vi "FiberWLCFruptCalc.vi"(9 "params in (all)":dbl[](array[numeric])=[0.0, 0.0, 6000.0, 50.0, 900.0, 197.0, 1.7, 0.3, 105.0, 80.0, 17.0, 5.0], 10 "tracename":string="E:\\users\\noort\\data\\270404\\_001.log") -> (1 "Channel data":dbl[][](array[numeric]), 2 "Channels":string[](array[string]), 3 "Lwrap (bp)":i16[](graph))   [LabVIEW 2018]
uses:
  <vilib>/Analysis/NI_AALBase.lvlib
panel:
  in  "Force treshold (pN)":dbl=5.0
  out "Lwrap (bp) 2":i32[](graph)
  out "F(z) Graph":cluster{"Data":dbl[], "Data":dbl[]}[](graph)
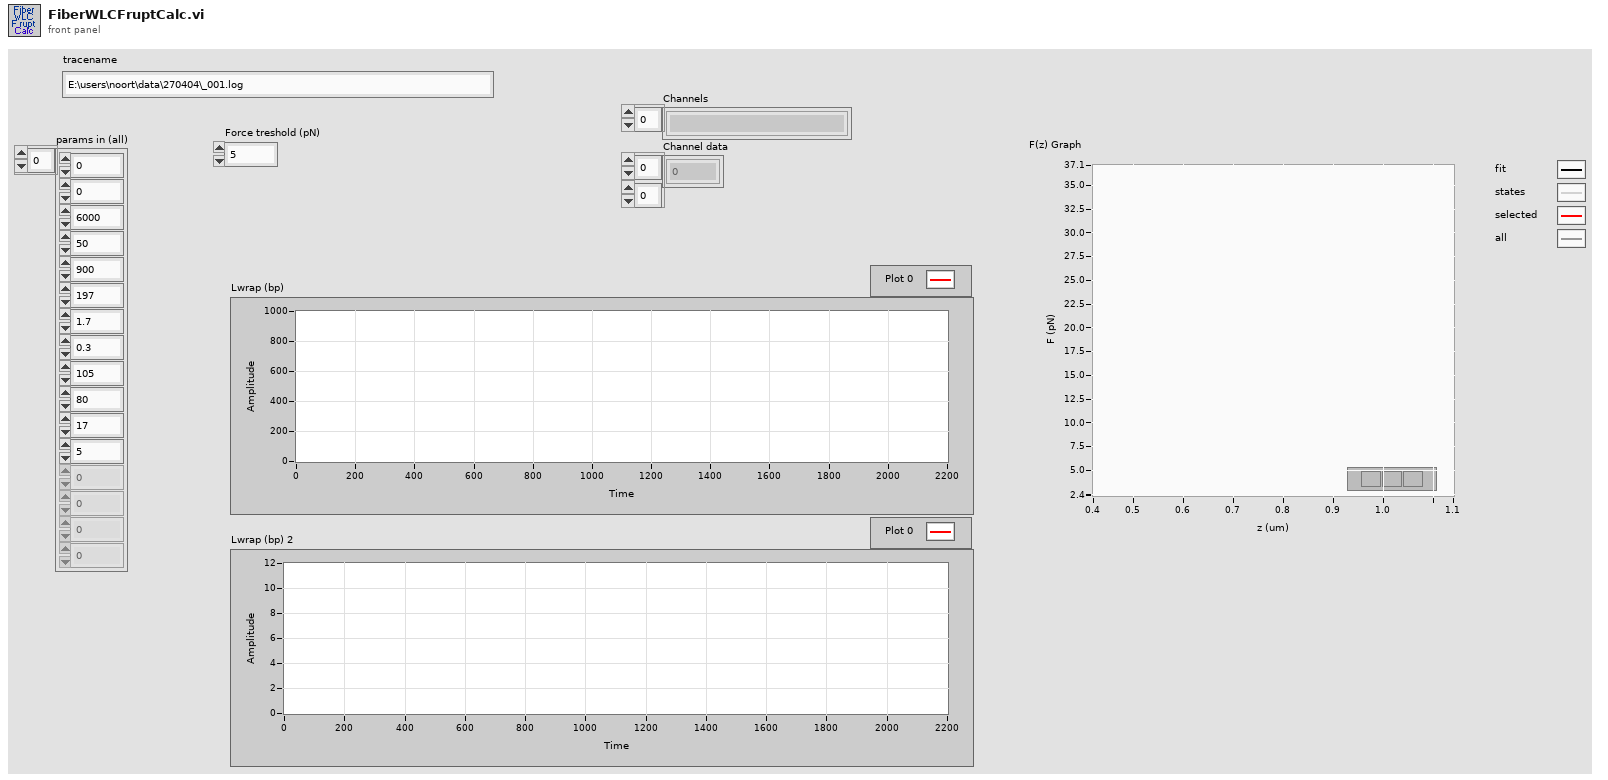
[diagram p1: front panel]
types:
  T1 = enum16{"Read", "Write", "Get channels", "Delete channels"}
  T2 = enum16{"Z0 (nm)", "dZ/dt (nm/s)", "L (bp)", "P (nm)", "S (pN)", "NRL (bp)", "NLD (nm)", "k (pN/nm)", "Lwrap1 (bp)", "Lwrap2 (bp)", "N4+N8", "N4"}
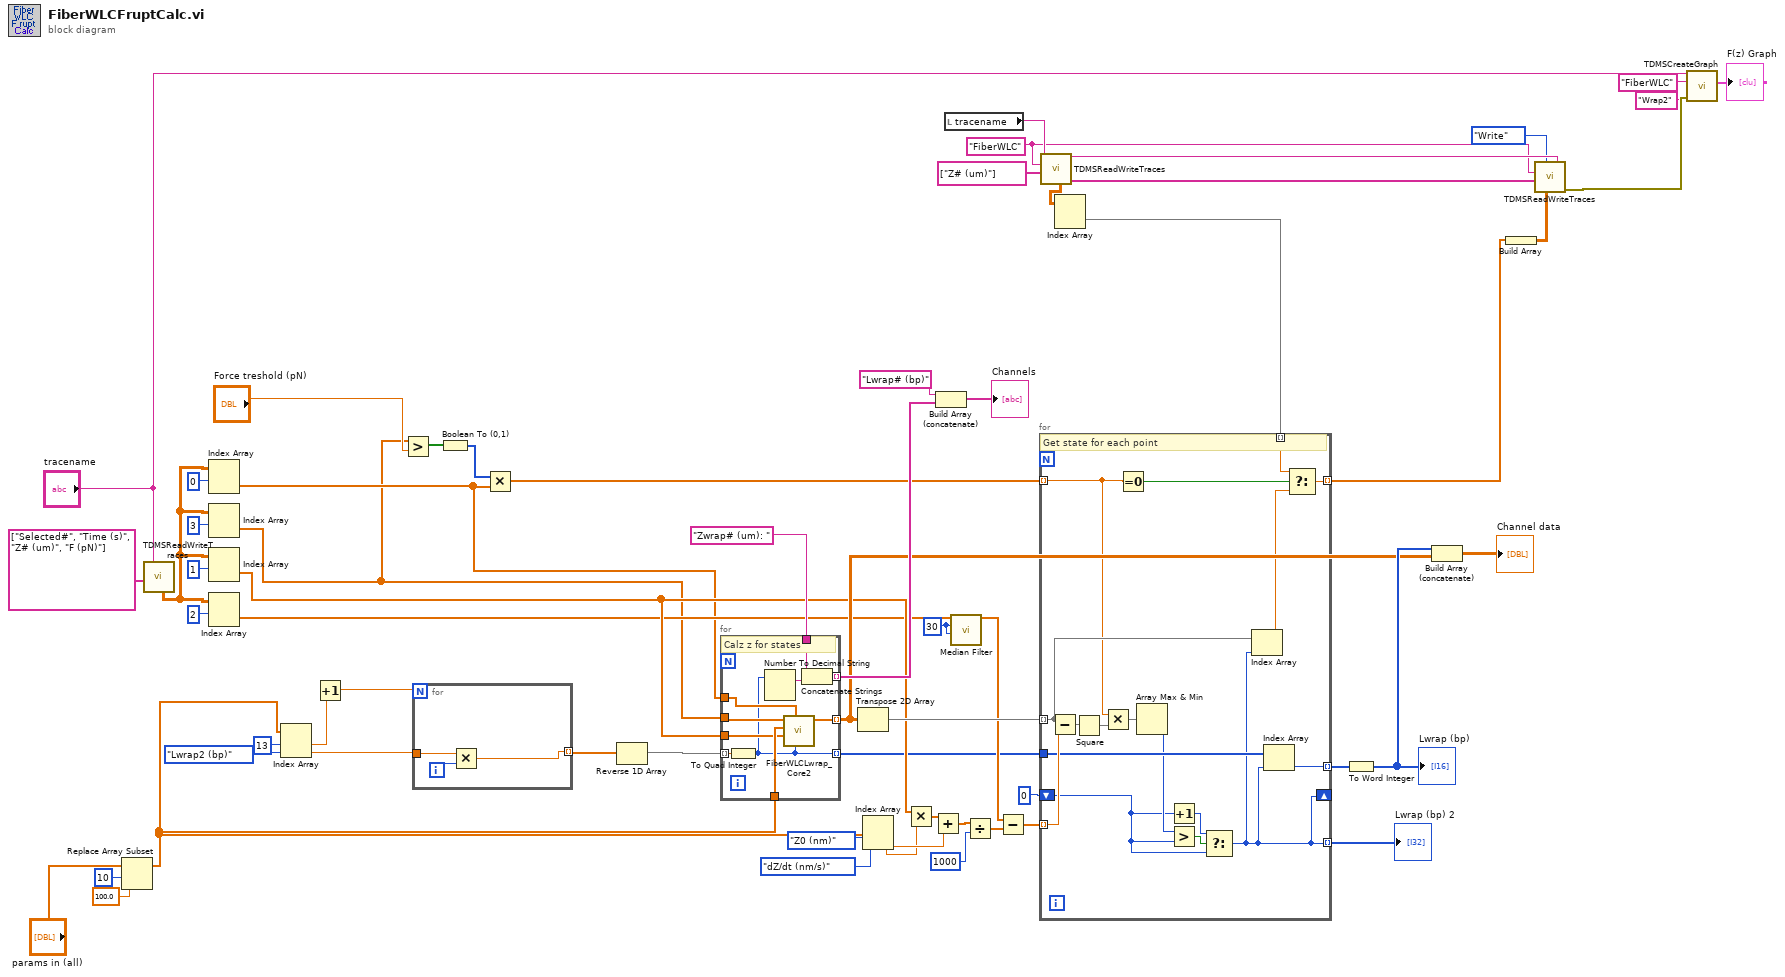
[diagram p0: block diagram]
diagram:
  w20 = "FiberWLC" ("group name")
  w32 = 30 ("left rank")
  n1 = Replace Array Subset(array="params in (all)", new element=100.0 ("new element/subarray"), index=10) -> (w1:dbl[])
  n2 = call "TDMSReadWriteTraces.vi"("Channels in"=string[] ["Selected#", "Time (s)", "Z# (um)", "F (pN)"] ("channel name(s) in"), "tracename"="tracename") -> ("Data out"=w55:dbl[][])  [unwired: 4 in, 5 out]
  n3 = Index Array(array=w55, index (row)=0) -> (element=w7:dbl[])  [unwired: 1 in]
  n4 = Index Array(array=w55, index (row)=3) -> (element=w6:dbl[])  [unwired: 1 in]
  n5 = Index Array(array=w55, index (row)=1) -> (element=w35:dbl[])  [unwired: 1 in]
  n6 = Index Array(array=w55, index (row)=2) -> (element=w34:dbl[])  [unwired: 1 in]
  n7 = Index Array(array=w1, index #1=13 ("index"), index #2=T2."Lwrap2 (bp)" ("Pars (Do not change)")) -> (element #1=w44:dbl, element #2=w42:dbl)
  n8 = Increment(x=w44) -> (x+1=w40:dbl)
  n9 = Greater?(x=w6, y="Force treshold (pN)") -> (0:w16:bool[])
  n10 = for {
    N: w40 -> [_]
    tunnel: w42 -> [w65]
    tunnel: [w64] -> w41 mode=indexing
    i -> [w66]
    n11 = Multiply(x=w65, y=w66) -> (x*y=w64:dbl)
  }
  n12 = Boolean To (0,1)(Boolean=w16) -> (0, 1=w15:i16[])
  n13 = Multiply(x=w15, y=w7) -> (x*y=w8:dbl[])
  n14 = Reverse 1D Array(array=w41) -> (reversed array=w29:dbl[])
  n15 = for {
    tunnel: w1 -> [w76]
    tunnel: w7 -> [w75]
    tunnel: w6 -> [w74]
    tunnel: w35 -> [w73]
    tunnel: [w72] -> w38 mode=indexing
    tunnel: w29 -> [w71] mode=indexing
    tunnel: [w70] -> w31 mode=indexing
    tunnel: "Zwrap# (um): " -> [w68]
    tunnel: [w67] -> w47 mode=indexing
    # "Calz z for states"
    n16 = To Quad Integer(1:w71) -> (0:w70:i64)
    n17 = Number To Decimal String(number=w70) -> (decimal integer string=w69:string)  [unwired: 1 in]
    n18 = call "FiberWLCLwrap_Core2.vi"("Lwrap"=w70, "selected (0,1)"=w75, "t (s)"=w73, "params in (all)"=w76, "F (pN)"=w74) -> ("z out (um)"=w72:dbl[])  [unwired: 3 in, 3 out]
    n19 = Concatenate Strings(w68, w69) -> (w67:string)
  }
  n20 = Transpose 2D Array(2D array=w38) -> (transposed array=w39:dbl[][])
  n21 = Index Array(array=w1, index #1=T2."Z0 (nm)" ("Pars (Do not change)"), index #2=T2."dZ/dt (nm/s)" ("Pars (Do not change)")) -> (element #1=w63:dbl, element #2=w61:dbl)
  n22 = Multiply(x=w35, y=w61) -> (x*y=w62:dbl[])
  n23 = Add(x=w62, y=w63) -> (x+y=w50:dbl[])
  n24 = Build Array (concatenate)("Lwrap# (bp)", w47) -> (→"Channels":string[])
  n25 = local read "tracename"() -> (w26:string)
  n26 = call <vilib>:"Median Filter.vi"("right rank"=w32, "left rank"=w32, "X"=w34) -> ("Filtered X"=w33:dbl[])  [unwired: 7 in, 1 out]
  n27 = Divide(x=w50, y=1000 ("width")) -> (x/y=w57:dbl[])
  n28 = Subtract(x=w33, y=w57) -> (x-y=w37:dbl[])
  n29 = call "TDMSReadWriteTraces.vi"("Channels in"=string[] ["Z# (um)"], "group name"=w20, "tracename"=w26) -> ("Channels out"=w23:string[], "tracename out"=w24:string, "Data out"=w25:dbl[][])  [unwired: 3 in, 3 out]
  n30 = Index Array(array=w25) -> (element=w19:dbl[])  [unwired: 2 in]
  n31 = for {
    tunnel: w39 -> [w87] mode=indexing
    tunnel: w37 -> [w93] mode=indexing
    tunnel: w31 -> [w92]
    tunnel: [w91] -> w30 mode=indexing
    tunnel: w8 -> [w86] mode=indexing
    shift-right: [w77] -> _
    shift-left: 0 -> [w78]
    tunnel: w19 -> [w84] mode=indexing
    tunnel: [w82] -> w9 mode=indexing
    tunnel: [w77] -> w5 mode=indexing
    # "Get state for each point"
    n32 = Subtract(x=w87, y=w93) -> (x-y=w88:dbl[])
    n33 = Square(x=w88) -> (x^2=w90:dbl[])
    n34 = Multiply(x=w86, y=w90) -> (x*y=w89:dbl[])
    n35 = Equal To 0?(x=w86) -> (x = 0?=w85:bool)
    n36 = Array Max & Min(array=w89) -> (min index (indices)=w81:i32)  [unwired: 3 out]
    n37 = Increment(x=w78) -> (x+1=w80:i32)
    n38 = Greater?(x=w81, y=w78) -> (0:w79:bool)
    n39 = Select(t=w80, s=w79, f=w78) -> (s? t:f=w77:i32)
    n40 = Index Array(array=w87, index=w77) -> (element=w83:dbl)
    n41 = Index Array(array=w92, index=w77) -> (element=w91:i64)
    n42 = Select(t=w84, s=w85, f=w83) -> (s? t:f=w82:dbl)
  }
  "Lwrap (bp) 2" <- w5
  n43 = To Word Integer(number=w30) -> (16bit integer=w48:i16[])
  "Lwrap (bp)" <- w48
  n44 = Build Array (concatenate)(w48, w38) -> (→"Channel data":dbl[][])
  n45 = Build Array(w9) -> (w22:dbl[][])
  n46 = call "TDMSReadWriteTraces.vi"("Data in"=w22, "Task"=T1."Write", "Channels in"=w23, "group name"=w20, "tracename"=w24) -> ("error out"=w12:errorcluster)  [unwired: 1 in, 5 out]
  n47 = call "TDMSCreateGraph.vi"("error in (no error)"=w12, "States"="Wrap2", "FitModel"="FiberWLC", "TraceName"="tracename") -> ("F(z) Graph"=→"F(z) Graph":cluster{"Data":dbl[], "Data":dbl[]}[])  [unwired: 5 in, 2 out]
